vi "State.Changed__LCR.vi"(5 "Data Changed?":bool, 7 "State Changed?":bool, 10 "Action in":T1 caption="Action In") -> (2 "Action":T1 caption="Action Out")   [LabVIEW 2011, in "BooleanXControl__LCR.xctl"]
doc: "Slimline interface to update the State and Data changed parts of teh action.\n\nORs the Action In with the Data\\State Changed? input."
uses:
  BooleanXControl__LCR.xctl
  <vilib>/_xctls/Action.ctl
  <vilib>/_xctls/XControlSupport.lvlib
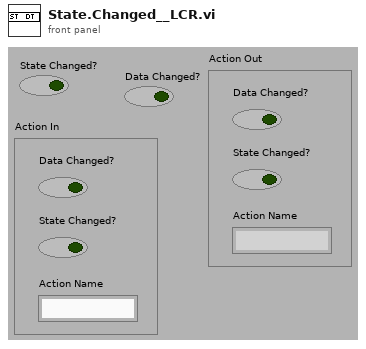
[diagram p1: front panel]
types:
  T1 = typedef "XControlSupport.lvlib/Action.ctl" = cluster{"Data Changed?":bool, "State Changed?":bool, "Action Name":string}
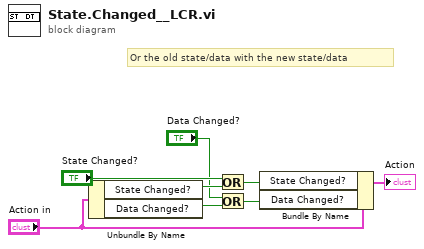
[diagram p0: block diagram]
diagram:
  # "Or the old state/data with the new state/data"
  n1 = Unbundle By Name("Action in") -> ("State Changed?"=w5:bool, "Data Changed?"=w2:bool)
  n2 = Or(x="State Changed?", y=w5) -> (x .or. y?=w8:bool)
  n3 = Or(x="Data Changed?", y=w2) -> (x .or. y?=w3:bool)
  n4 = Bundle By Name(cluster="Action in", "State Changed?"=w8, "Data Changed?"=w3) -> (→"Action":T1)
